vi "Sychronous Odometry Processor.vi"(8 "error in (no error)":errorcluster, 10 "Encoder Data":T1, 11 "Heading":T2) -> (0 "error out":errorcluster, 3 "Reset?":bool)   [LabVIEW 2018]
uses:
  ADIS16470/Typedef/ADIS16470 Data.ctl
  Typedef/Odometry.ctl
  <vilib>/Analysis/coordinate.llb/2D Cartesian Coordinate Rotation.vi
  <vilib>/Analysis/coordinate.llb/2D Cartesian Coordinate Rotation (Scalar).vi
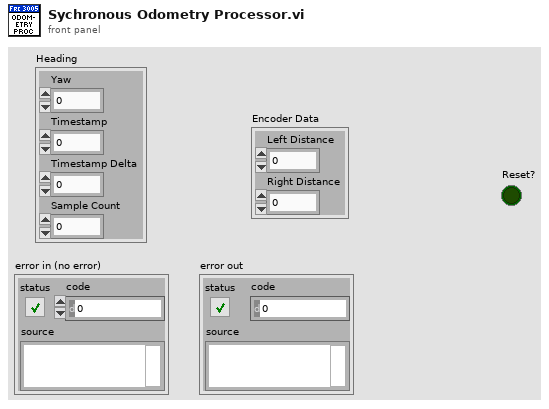
[diagram p1: front panel]
types:
  T1 = cluster{"Left Distance":dbl, "Right Distance":dbl}
  T2 = typedef "ADIS16470 Data.ctl" = cluster{"Yaw":dbl, "Timestamp":dbl, "Timestamp Delta":dbl, "Sample Count":u16}
  T3 = typedef "Odometry.ctl" = cluster{"x":dbl, "y":dbl, "theta":dbl, "Left Encoder":dbl, "Right Encoder":dbl, "Late Iterations":i16}
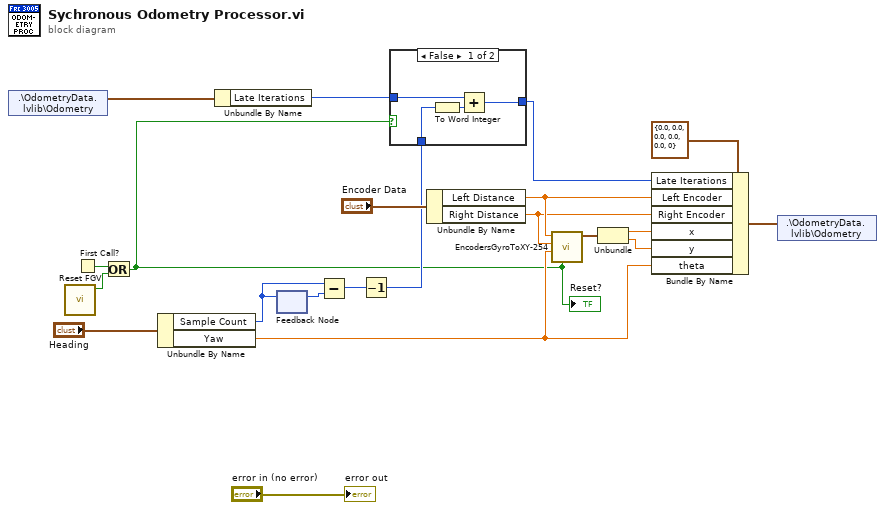
[diagram p0: block diagram]
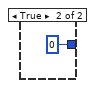
[diagram p2: hidden frame]
diagram:
  n1 = shared-variable ".\\OdometryData.lvlib\\Odometry"() -> (w5:T3)  [unwired: 1 in, 1 out]
  n2 = call "Reset FGV.vi"() -> ("Reset?"=w12:bool)  [unwired: 11 in]
  n3 = First Call?() -> (First Call?: T/F=w13:bool)
  n4 = Or(x=w13, y=w12) -> (x .or. y?=w1:bool)
  "Reset?" <- w1
  n5 = Unbundle By Name("Heading") -> ("Sample Count"=w7:u16, "Yaw"=w14:dbl)
  n6 = Unbundle By Name(w5) -> ("Late Iterations"=w4:i16)
  n7 = feedback-in #1(w7) -> ()
  n8 = feedback #1() -> (w8:u16)  [unwired: 1 in]
  n9 = Subtract(x=w7, y=w8) -> (x-y=w6:u16)
  n10 = Decrement(x=w6) -> (x-1=w3:u16)
  n11 = case shown="False" w1 {
    tunnel: w4 -> [w25 _]
    tunnel: w3 -> [w24 _]
    tunnel: [w23 i16 0] -> w2
    frame False {
      n12 = To Word Integer(number=w24) -> (16bit integer=w22:i16)
      n13 = Add(x=w25, y=w22) -> (x+y=w23:i16)
    }
    frame True {
    }
  }
  n14 = Unbundle By Name("Encoder Data") -> ("Left Distance"=w10:dbl, "Right Distance"=w9:dbl)
  n15 = call "EncodersGyroToXY-254.vi"("Reset"=w1, "Angle (degrees)"=w14, "Right Distance"=w9, "Left Distance"=w10) -> ("Location"=w17:cluster{"X":dbl, "Y":dbl})  [unwired: 7 in]
  n16 = Unbundle(w17) -> ("X"=w16:dbl, "Y"=w15:dbl)
  n17 = Bundle By Name(cluster=T3 {"x"=0.0, "y"=0.0, "theta"=0.0, "Left Encoder"=0.0, "Right Encoder"=0.0, "Late Iterations"=0} ("Odometry"), "Late Iterations"=w2, "Left Encoder"=w10, "Right Encoder"=w9, "x"=w16, "y"=w15, "theta"=w14) -> (w20:T3)
  n18 = shared-variable ".\\OdometryData.lvlib\\Odometry"(w20) -> ()  [unwired: 1 in, 1 out]
  "error out" <- "error in (no error)"
